vi "Meas Check Sequence Files.vi"(8 "error in":errorcluster, 10 "don't ask (False)":bool, 11 "sequence setup":T1) -> (0 "error out":errorcluster, 2 "cancel?":bool, 3 "sequence setup out (copy)":T1)   [LabVIEW 2018]
doc: "This VI will check if there are some files with filenames that collides with file name base of the new measurement. If so, it will as operator to either remove them or cancel. This panel can be ihibited as option, but it will still ask if some non-expected files are found in the path. This is kind of protection against accidental erase of invalid path."
uses:
  Meas Sequence Configuration.ctl
  Meas Sampling Configuration.ctl
  adc/ADC Trig Config.ctl
  adc/ADC Trig Mode Source.ctl
  adc/ADC Trig Coupling.ctl
  adc/ADC Trig Slope.ctl
  processing/QWTB/Meas Proc QWTB Algorithm Parameter Data.ctl
  Meas Range Mode.ctl
  Meas Sampling Rate Mode.ctl
  other/GUI Panel Control Action.ctl
  varilib/varilib.lvlib
panel:
  in  "btn cancel":bool
  in  "btn rem":bool
  out "Files to remove":string
  # "Following existing files collides with the new measurement file names.\nDo you want to REMOVE them or CANCEL the operation and change file names?"
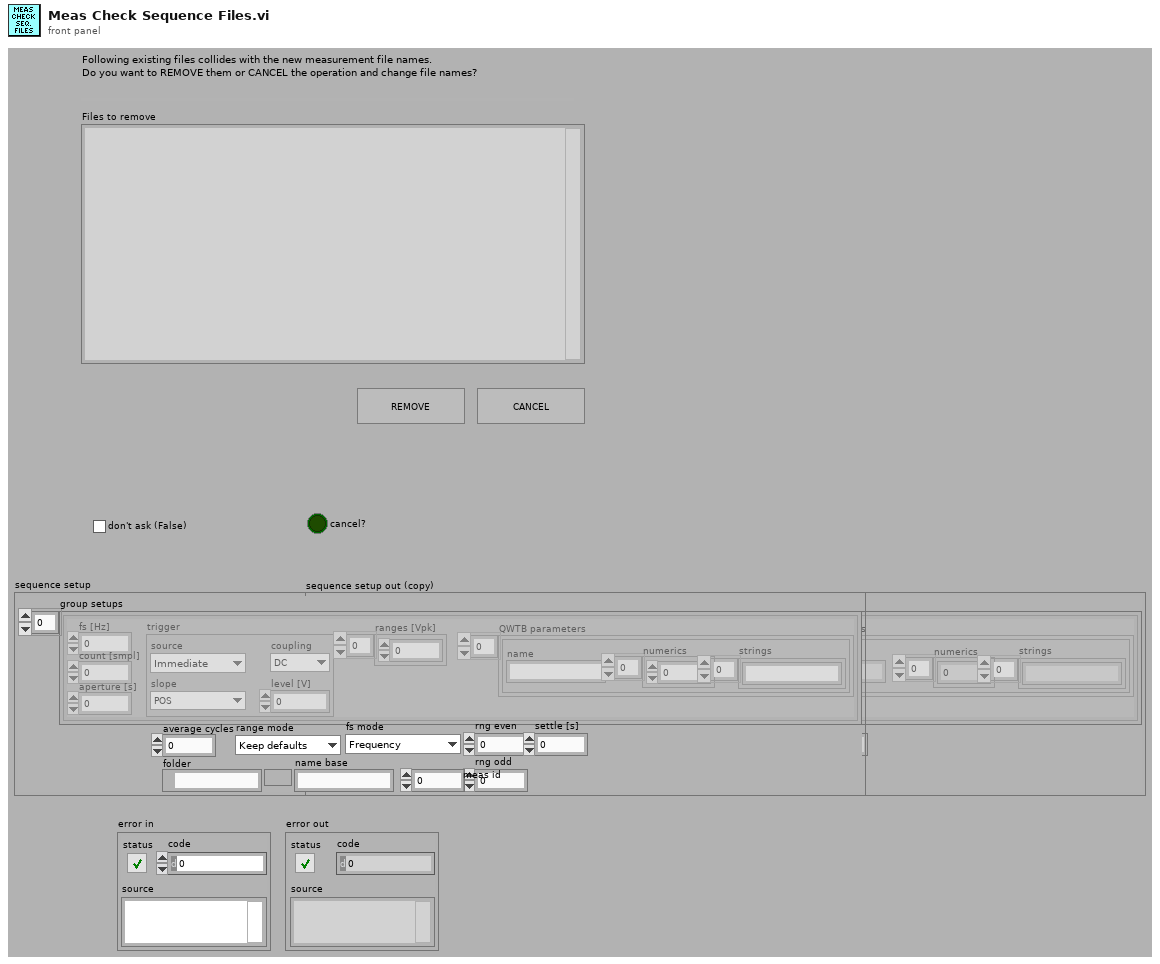
[diagram p1: front panel]
types:
  T1 = typedef "Meas Sequence Configuration.ctl" = cluster{"group setups":T2[], "average cycles":i32, "range mode":T8, "fs mode":T9, "rng even":dbl, "rng odd":dbl, "folder":path, "name base":string, "meas id":i32, "settle [s]":dbl}
  T2 = typedef "Meas Sampling Configuration.ctl" = cluster{"fs [Hz]":dbl, "count [smpl]":i64, "aperture [s]":dbl, "trigger":T3, "ranges [Vpk]":dbl[], "QWTB parameters":T7[]}
  T3 = typedef "ADC Trig Config.ctl" = cluster{"source":T4, "level [V]":dbl, "coupling":T5, "slope":T6}
  T4 = typedef "ADC Trig Mode Source.ctl" = enum16{"Immediate", "External", "Level"}
  T5 = typedef "ADC Trig Coupling.ctl" = enum16{"DC", "AC"}
  T6 = typedef "ADC Trig Slope.ctl" = enum16{"POS", "NEG"}
  T7 = typedef "Meas Proc QWTB Algorithm Parameter Data.ctl" = cluster{"name":string, "numerics":dbl[], "strings":string[]}
  T8 = typedef "Meas Range Mode.ctl" = enum16{"Keep defaults", "Set All channels", "Set Odd and Even channels"}
  T9 = typedef "Meas Sampling Rate Mode.ctl" = enum16{"Frequency", "Period"}
  T10 = typedef "GUI Panel Control Action.ctl" = enum16{"Open panel", "Close panel", "Bring To Front"}
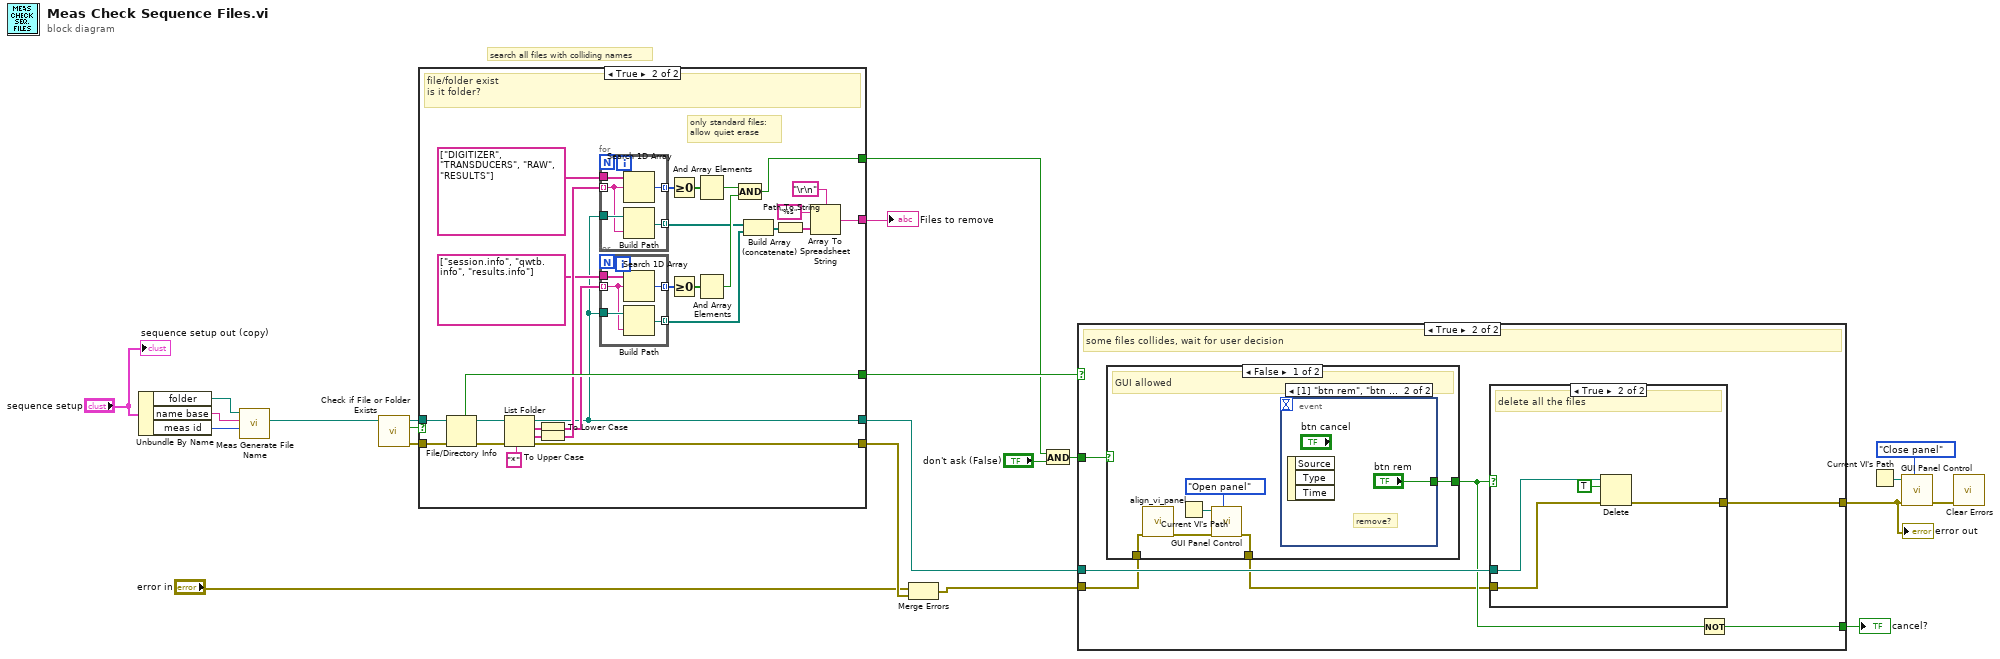
[diagram p0: block diagram]
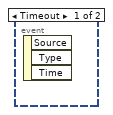
[diagram p4: hidden frame]
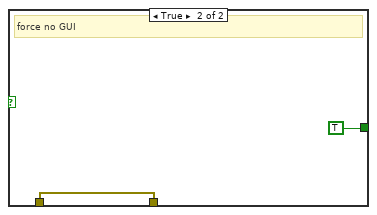
[diagram p5: hidden frame]
diagram:
  # "search all files with colliding names"
  n1 = Unbundle By Name("sequence setup") -> ("folder"=w20:path, "name base"=w19:string, "meas id"=w18:i32)
  n2 = call "Meas Generate File Name.vi"("meas id"=w18, "name base"=w19, "folder"=w20) -> ("measurement root folder"=w17:path)  [unwired: 4 in, 4 out]
  n3 = call <vilib>:"Check if File or Folder Exists.vi"("path"=w17) -> ("error out"=w15:errorcluster, "file or folder exists?"=w14:bool, "dup path"=w16:path)  [unwired: 8 in]
  n4 = case shown="True" w14 {
    tunnel: w16 -> [w23 w52]
    tunnel: w15 -> [w24 w51]
    tunnel: [_ w50] -> w12
    tunnel: [w24 w46] -> w13
    tunnel: [w23 w33] -> w10
    tunnel: [_ w26] -> w9
    tunnel: [_ w25] -> w7
    frame False {
    }
    frame True {
      # "only standard files:\nallow quiet erase"
      # "file/folder exist\nis it folder?"
      n5 = File/Directory Info(path=w52, error in=w51) -> (path out=w49:path, directory=w50:bool, error out=w48:errorcluster)  [unwired: 4 out]
      n6 = List Folder(path=w49, pattern="*", error in=w48) -> (path out=w33:path, filenames=w37:string[], folder names=w45:string[], error out=w46:errorcluster)  [unwired: 1 in]
      n7 = To Lower Case(string=w37) -> (all lower case string=w36:string[])
      n8 = To Upper Case(1:w45) -> (0:w44:string[])
      n9 = for {
        tunnel: w44 -> [w59] mode=indexing
        tunnel: string[] ["DIGITIZER", "TRANSDUCERS", "RAW", "RESULTS"] -> [w62]
        tunnel: [w61] -> w42 mode=indexing
        tunnel: w33 -> [w60]
        tunnel: [w58] -> w32 mode=indexing
        n10 = Search 1D Array(1D array=w62, element=w59) -> (index of element=w61:i32)  [unwired: 1 in]
        n11 = Build Path(base path=w60, name or relative path=w59) -> (appended path=w58:path)
      }
      n12 = for {
        tunnel: w36 -> [w54] mode=indexing
        tunnel: string[] ["session.info", "qwtb.info", "results.info"] -> [w57]
        tunnel: [w56] -> w39 mode=indexing
        tunnel: w33 -> [w55]
        tunnel: [w53] -> w31 mode=indexing
        n13 = Search 1D Array(1D array=w57, element=w54) -> (index of element=w56:i32)  [unwired: 1 in]
        n14 = Build Path(base path=w55, name or relative path=w54) -> (appended path=w53:path)
      }
      n15 = Greater Or Equal To 0?(x=w42) -> (x >= 0?=w41:bool[])
      n16 = Greater Or Equal To 0?(x=w39) -> (x >= 0?=w40:bool[])
      n17 = And Array Elements(Boolean array=w41) -> (logical AND=w35:bool)
      n18 = And Array Elements(Boolean array=w40) -> (logical AND=w34:bool)
      n19 = Compound Arithmetic op=AND(w35, w34) -> (w25:bool)
      n20 = Build Array (concatenate)(w32, w31) -> (w30:path[])
      n21 = Path To String(path=w30) -> (string=w29:string[])
      n22 = Array To Spreadsheet String(delimiter (Tab)="\r\n", array=w29, 3:"%s" ("format string")) -> (spreadsheet string=w26:string)
    }
  }
  "Files to remove" <- w9
  n23 = Merge Errors("error in", w13) -> (w11:errorcluster)
  n24 = Compound Arithmetic op=AND(w7, "don't ask (False)") -> (w6:bool)
  n25 = case shown="True" w12 {
    tunnel: w10 -> [_ w70]
    tunnel: w11 -> [w63 w65]
    tunnel: [w63 w66] -> w2
    tunnel: [_ w69] -> w21
    tunnel: w6 -> [_ w67]
    frame False {
      # "no files collides, go away"
    }
    frame True {
      # "some files collides, wait for user decision"
      n26 = case shown="False" w67 {
        tunnel: [w76 TRUE] -> w68
        tunnel: w65 -> [w72 w78]
        tunnel: [w71 w78] -> w64
        frame False {
          # "GUI allowed"
          n27 = call "align_vi_panel.vi"("error in"=w72) -> ("error out"=w73:errorcluster)  [unwired: 10 in]
          n28 = Current VI's Path() -> (path=w74:path)
          n29 = call "GUI Panel Control.vi"("action (open panel)"=GUI_Panel_Control_Action."Open panel", "error in (no error)"=w73, "vi path"=w74) -> ("error out"=w71:errorcluster)  [unwired: 8 in]
          n30 = event shown="[1] \"btn rem\", \"btn cancel\": Value Change;  Panel Close" {
            selector: _ -> [_ _]
            dyn-events: _ -> [_ _]
            timeout: _ -> [_ _]
            tunnel: [_ "btn rem"] -> w76
            event Timeout {
              n31 = event-data() -> ()  [unwired: 1 in, 3 out]
            }
            event "btn rem", "btn cancel": Value Change; Panel Close {
              # "remove?"
              n32 = event-data() -> ()  [unwired: 1 in, 3 out]
            }
          }
        }
        frame True {
          # "force no GUI"
        }
      }
      n33 = case shown="True" w68 {
        tunnel: w70 -> [_ w84]
        tunnel: w64 -> [w80 w83]
        tunnel: [w80 w82] -> w66
        frame False {
        }
        frame True {
          # "delete all the files"
          n34 = Delete(path (use dialog)=w84, entire hierarchy (F)=TRUE, error in=w83) -> (error out=w82:errorcluster)  [unwired: 2 in, 2 out]
        }
      }
      n35 = Not(x=w68) -> (.not. x?=w69:bool)
    }
  }
  "error out" <- w2
  "cancel?" <- w21
  n36 = Current VI's Path() -> (path=w3:path)
  n37 = call "GUI Panel Control.vi"("action (open panel)"=GUI_Panel_Control_Action."Close panel", "error in (no error)"=w2, "vi path"=w3) -> ("error out"=w1:errorcluster)  [unwired: 8 in]
  n38 = call <vilib>:"Clear Errors.vi"("error in (no error)"=w1) -> ()  [unwired: 5 in, 2 out]
  "sequence setup out (copy)" <- "sequence setup"
